vi "move_in_horizontal_plain.vi"(5 "direction":bool, 6 "Echo Mode":i32, 7 "Unit of Move":T1 items=["STEPS", "MICRONS / DEG", "CENTIMETER / DEG", "INCHES / DEG"], 8 "error in (no error)":errorcluster, 9 "Speed [micron/s]":dbl=750.0, 10 "Steps":dbl format="%#_13g", 11 "ComPort":refnum<visa-resource-name>="COM16") -> (0 "error out":errorcluster={"status"=FALSE, "code"=1073676294, "source"="VISA Read in write_read.vi"}, 1 "move time (ms)":u32, 2 "actual angle":dbl format="%_6g", 3 "VISA ressource out":refnum<visa-resource-name>)   [LabVIEW 2018]
uses:
  Units_of_Move.ctl
  ConversionAndInformation/Unit_Control.ctl
  MCode_LV_86/Set Parameter.ctl
panel:
  out "steps motor 1 ()":string
  out "steps motor 2 ()":string
  out "move time (ms) 2":u32
  out "move time (ms) 1":u32
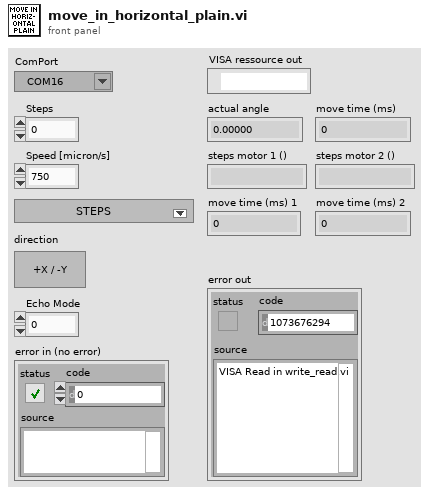
[diagram p1: front panel]
types:
  T1 = typedef "Units_of_Move.ctl" = u16
  T2 = typedef "Set Parameter.ctl" = enum16{"Acceleration (A)", "Baud Rate (BD)", "Counter 1 (C1)", "Counter 2 (C2)", "Control C Software Reset (CE)", "Check Sum Enable (CK)", "Clock Mode (CM)", "Clock Mode Ratio (CR)", "Clock Mode Out Step Width (CW)", "Deceleration (D)", "Digital Filtering, Input 1 (D1)", "Digital Filtering, Input 2 (D2)", "Digital Filtering, Input 3 (D3)", "Digital Filtering, Input 4 (D4)", "Digital Filtering, Input 5 (D5)", "Digital Filtering, Input 9 (D9)", "Digital Filtering, Input 10 (D10)", "Digital Filtering, Input 11 (D11)", "Digital Filtering, Input 12 (D12)", "Deadband (DB)", "Decrement Variable (DC)", "Enable/Disable Drive (DE)", "Device Name (DN)", "End Program Execution (E)", "Encoder Function Enable (EE)", "Error Flag (EF)", "Encoder Lines (EL)", "Echo Mode (EM)", "Error Value (ER)", "Escape (ES)", "Execute Program at Address (EX)", "Firmware Version (VR)", "Hold (H)", "Hold Current (HC)", "Hold Current Delay Time (HI)", "Home to Encoder Index (HM)", "Home to Home Switch (HT)", "Increment Variable (IC)", "Initialize Parameters to NVM (IP)", "Input into Variable (IV)", "Jog Enable (JE)", "Limit Stop Mode (LM)", "Move Absolute (MA)", "Move Relative (MR)", "MicroStepping Select (MS)", "Motor Settling Delay Time (MT)", "Moving [Flag] (MV)", "Output 1 (O1)", "Output 2 (O2)", "Output 3 (O3)", "Output 4 (O4)", "Output 9 (O9)", "Output 10 (O10)", "Output 11 (O11)", "Output 12 (O12)", "Output High Byte (9-12) (OH)", "Output Low Byte (1-4) (OL)", "Output Total (1-4 and 9-12) (OT)", "Position (P)", "Position Maintenance (PM)", "Party Mode (PY)", "Register 1 (R1)", "Register 2 (R2)", "Register 3 (R3)", "Register 4 (R4)", "Reset Error(\\03)", "Run Current (RC)", "Stall Factor (SF)", "Slew (SL)", "Stall Mode Set (SM)", "Upgrade Firmware (UG)", "Velocity Initial (VI)", "Velocity Maximum (VM)", "Current1 (I1)", "Current2 (I2)", "Current3 (I3)", "Current4 (I4)", "Current5 (I5)", "Current6 (I6)", "Save (S)"}
  T3 = typedef "Unit_Control.ctl" = enum16{"Angle (Degrees)", "Rad", "Angle [TMC]", "Microsteps [TMC]", "Inches", "Nanometer", "Meter", "Centimeter", "Millimeter", "Micron"}
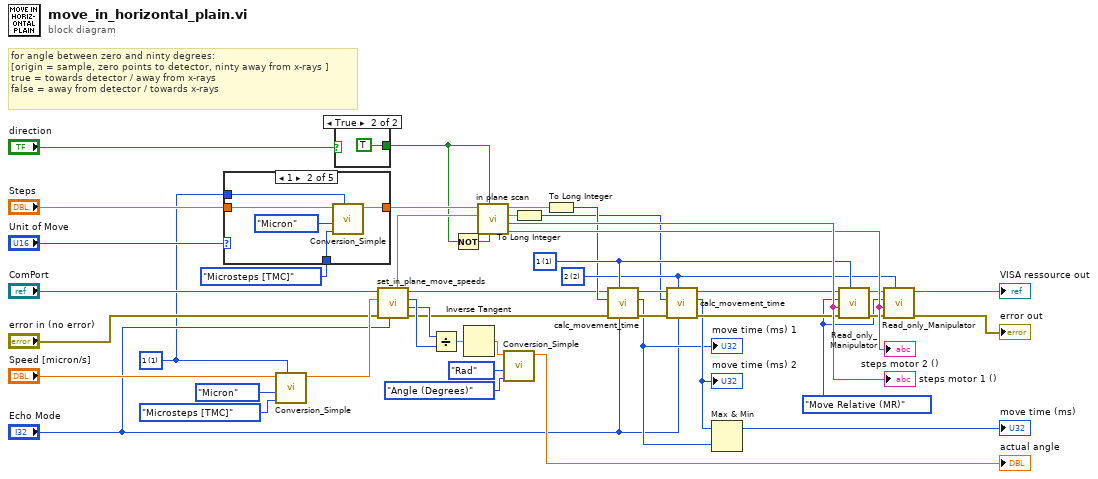
[diagram p0: block diagram]
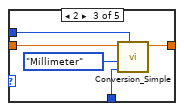
[diagram p3: hidden frame]
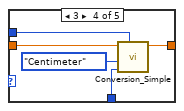
[diagram p4: hidden frame]
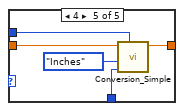
[diagram p5: hidden frame]
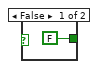
[diagram p6: hidden frame]
diagram:
  w2 = Set_Parameter."Move Relative (MR)" ("Command")
  w1 = u16 1 items=["none", "1", "2", "3", "4", "all"] ("Motor")
  w39 = u16 1 items=["none", "1", "2", "3", "4", "all"] ("Motor")
  w38 = u16 2 items=["none", "1", "2", "3", "4", "all"] ("Motor")
  # "for angle between zero and ninty degrees:\n[origin = sample, zero points to detector, ninty away from x-rays ]\ntrue = towards detector / away from x-rays\nfalse = away from detector / towards x-rays"
  n1 = case shown="1" "Unit of Move" {
    tunnel: Unit_Control."Microsteps [TMC]" ("Input Unit") -> [_ w50 w55 w60 w65]
    tunnel: [w46 w49 w54 w59 w64] -> w14
    tunnel: "Steps" -> [w46 w48 w53 w58 w63]
    tunnel: w1 -> [_ w47 w52 w57 w62]
    frame 0, Default {
    }
    frame 1 {
      n2 = call "Conversion_Simple.vi"("Motor"=w47, "Output Unit"=w50, "Input Unit"=Unit_Control."Micron", "Input"=w48) -> ("Output"=w49:dbl)  [unwired: 6 in, 1 out]
    }
    frame 2 {
      n3 = call "Conversion_Simple.vi"("Motor"=w52, "Output Unit"=w55, "Input Unit"=Unit_Control."Millimeter", "Input"=w53) -> ("Output"=w54:dbl)  [unwired: 6 in, 1 out]
    }
    frame 3 {
      n4 = call "Conversion_Simple.vi"("Motor"=w57, "Output Unit"=w60, "Input Unit"=Unit_Control."Centimeter", "Input"=w58) -> ("Output"=w59:dbl)  [unwired: 6 in, 1 out]
    }
    frame 4 {
      n5 = call "Conversion_Simple.vi"("Motor"=w62, "Output Unit"=w65, "Input Unit"=Unit_Control."Inches", "Input"=w63) -> ("Output"=w64:dbl)  [unwired: 6 in, 1 out]
    }
  }
  n6 = call "Conversion_Simple.vi"("Motor"=w1, "Output Unit"=Unit_Control."Microsteps [TMC]" ("Input Unit"), "Input Unit"=Unit_Control."Micron", "Input"="Speed [micron/s]") -> ("Output"=w20:dbl)  [unwired: 6 in, 1 out]
  n7 = case shown="True" "direction" {
    tunnel: [FALSE ("invert x") TRUE ("invert x")] -> w8
    frame False {
    }
    frame True {
    }
  }
  n8 = call "set_in_plane_move_speeds.vi"("Echo Mode"="Echo Mode", "error in (no error)"="error in (no error)", "V_max total"=w20, "VISA resource name"="ComPort") -> ("error out"=w5:errorcluster, "V_max Motor 2"=w19:i32, "V_max Motor 1"=w22:i32, "VISA ressource out"=w18:refnum<visa-resource-name>, "Angle Sample Holder"=w21:dbl)  [unwired: 3 in]
  n9 = Divide(x=w19, y=w22) -> (x/y=w31:dbl)
  n10 = Not(x=w8) -> (.not. x?=w32:bool)
  n11 = Inverse Tangent(1:w31) -> (0:w30:dbl)
  n12 = call "in plane scan.vi"("invert y"=w32, "invert x"=w8, "angle (degrees)"=w21, "v total"=w14) -> ("v_y string"=w43:string, "v_x string"=w44:string, "v_y"=w35:dbl, "v_x"=w37:dbl)  [unwired: 2 in, 2 out]
  "steps motor 1 ()" <- w44
  "steps motor 2 ()" <- w43
  n13 = call "Conversion_Simple.vi"("Output Unit"=Unit_Control."Angle (Degrees)", "Input Unit"=Unit_Control."Rad", "Input"=w30) -> ("Output"=→"actual angle":dbl)  [unwired: 7 in, 1 out]
  n14 = To Long Integer(number=w35) -> (32bit integer=w34:i32)
  n15 = To Long Integer(number=w37) -> (32bit integer=w36:i32)
  n16 = call "calc_movement_time.vi"("Echo Mode"="Echo Mode", "Motor"=w39, "error in (no error)"=w5, "steps"=w36, "VISA ressource in"=w18) -> ("error out"=w42:errorcluster, "move time (ms)"=w24:u32, "VISA ressource out"=w41:refnum<visa-resource-name>)  [unwired: 3 in, 1 out]
  "move time (ms) 1" <- w24
  n17 = call "calc_movement_time.vi"("Echo Mode"="Echo Mode", "Motor"=w38, "error in (no error)"=w42, "steps"=w34, "VISA ressource in"=w41) -> ("error out"=w26:errorcluster, "move time (ms)"=w25:u32, "VISA ressource out"=w40:refnum<visa-resource-name>)  [unwired: 3 in, 1 out]
  "move time (ms) 2" <- w25
  n18 = Max & Min(x=w25, y=w24) -> (max(x,y)=→"move time (ms)":u32)  [unwired: 1 out]
  n19 = call "Read_only_Manipulator.vi"("Motor"=w39, "error in (no error)"=w26, "Value"=w44, "Command"=w2, "VISA resource name"=w40) -> ("error out"=w3:errorcluster, "VISA ressource out"=w4:refnum<visa-resource-name>)  [unwired: 3 in, 2 out]
  n20 = call "Read_only_Manipulator.vi"("Motor"=w38, "error in (no error)"=w3, "Value"=w43, "Command"=w2, "VISA resource name"=w4) -> ("error out"=→"error out":errorcluster, "VISA ressource out"=→"VISA ressource out":refnum<visa-resource-name>)  [unwired: 3 in, 2 out]
